vi "util_SwitchableDevice_cls_Get Device State.vi"(0 "Interface_object in":refnum<class>, 5 "error in (no error)":errorcluster) -> (14 "Interface_object out":refnum<class>, 17 "Device State":bool, 19 "error out":errorcluster)   [LabVIEW 2018, in "Lamp.lvclass"]
uses:
  Lamp.lvclass
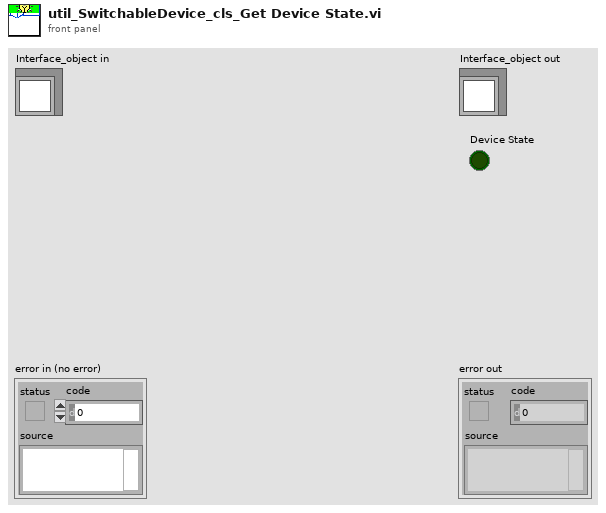
[diagram p1: front panel]
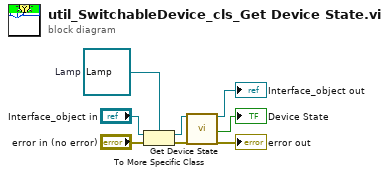
[diagram p0: block diagram]
diagram:
  w7 = refnum<class "Lamp.lvclass"> refnum  # Lamp
  n1 = To More Specific Class(target class=w7, reference="Interface_object in", error in="error in (no error)") -> (specific class reference=w5:refnum<class "Lamp.lvclass">, error out=w6:errorcluster)
  n2 = call-dynamic "Get Device State.vi"("Interface_object in"=w5, "error in (no error)"=w6) -> ("Interface_object out"=→"Interface_object out":refnum<class "Lamp.lvclass">, "Device State"=→"Device State":bool, "error out"=→"error out":errorcluster)  [unwired: 15 in]
